vi "TestDBCommands.vi"() -> ()   [LabVIEW 2012]
uses:
  <vilib>/addons/database/Connection.llb/DB Tools Open Connec (Path).vi
  <vilib>/addons/database/Connection.llb/Conn Execute.vi
  <vilib>/addons/database/Recordset.llb/Rec Fetch Recordset Data (R).vi
  <vilib>/addons/database/Recordset.llb/Rec Destroy - Connection.vi
  <vilib>/addons/database/Auxilliary.llb/DB Tools Parameter Dir.ctl
  <vilib>/addons/database/NI_Database_API.lvlib
  <vilib>/addons/database/Auxilliary.llb/DB Tools DataTypes.ctl
  <vilib>/addons/database/Auxilliary.llb/DB Tools Parameter Info.ctl
  <vilib>/addons/database/Command.llb/Cmd Set Parameter Value (C).vi
  <vilib>/addons/database/Command.llb/Cmd Execute.vi
  <vilib>/addons/database/Recordset.llb/Rec Destroy - Command.vi
  <vilib>/addons/database/Command.llb/Cmd Delete.vi
  Controls/ProbeStationId.vi
panel:
  out "SameId?":bool
  out "Tested?":bool
  out "Exists?":bool
  in  "Type":string
  out "String":string
  out "error out":errorcluster
  in  "WaferId":string
  in  "connection":path
  in  "error IO":errorcluster
  out "System":string
  out "Run Number":string
  out "Pocket":string
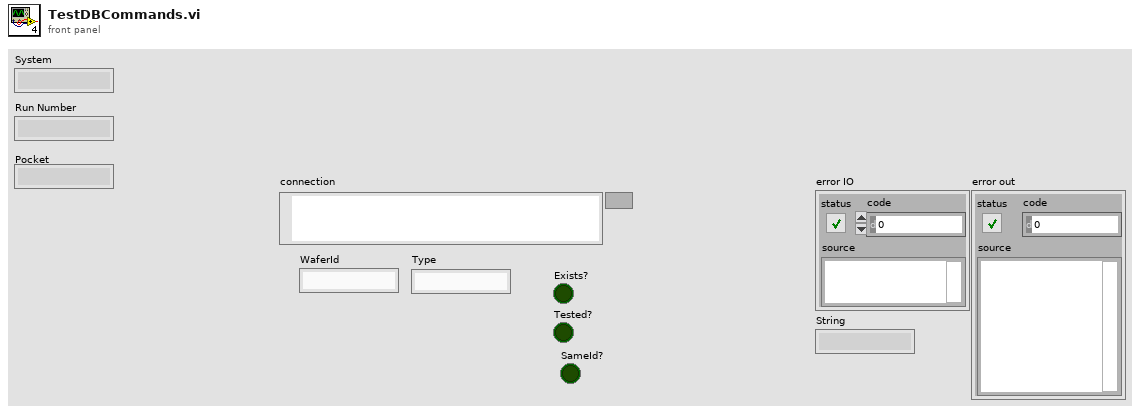
[diagram p1: front panel]
types:
  T1 = typedef "NI_Database_API.lvlib/DB Tools Parameter Info.ctl" = cluster{"parameter name":string, "type":T2, "direction":T3, "value":variant}
  T2 = typedef "NI_Database_API.lvlib/DB Tools DataTypes.ctl" = enum16{"String", "Long (I32)", "Single (SGL)", "Double (DBL)", "Date/Time", "Binary"}
  T3 = typedef "NI_Database_API.lvlib/DB Tools Parameter Dir.ctl" = enum32{"Input", "Output", "Input/Output", "Return Value"}
  T4 = typedef "NI_Database_API.lvlib/Conn ObjectReference.ctl" = refnum<k1>
  T5 = typedef "NI_Database_API.lvlib/Cmd ObjectReference.ctl" = refnum<k1>
  T6 = typedef "NI_Database_API.lvlib/Cmd-Rec Object Reference.ctl" = refnum<k1>
  T7 = typedef "NI_Database_API.lvlib/Rec ObjectReference.ctl" = refnum<k1>
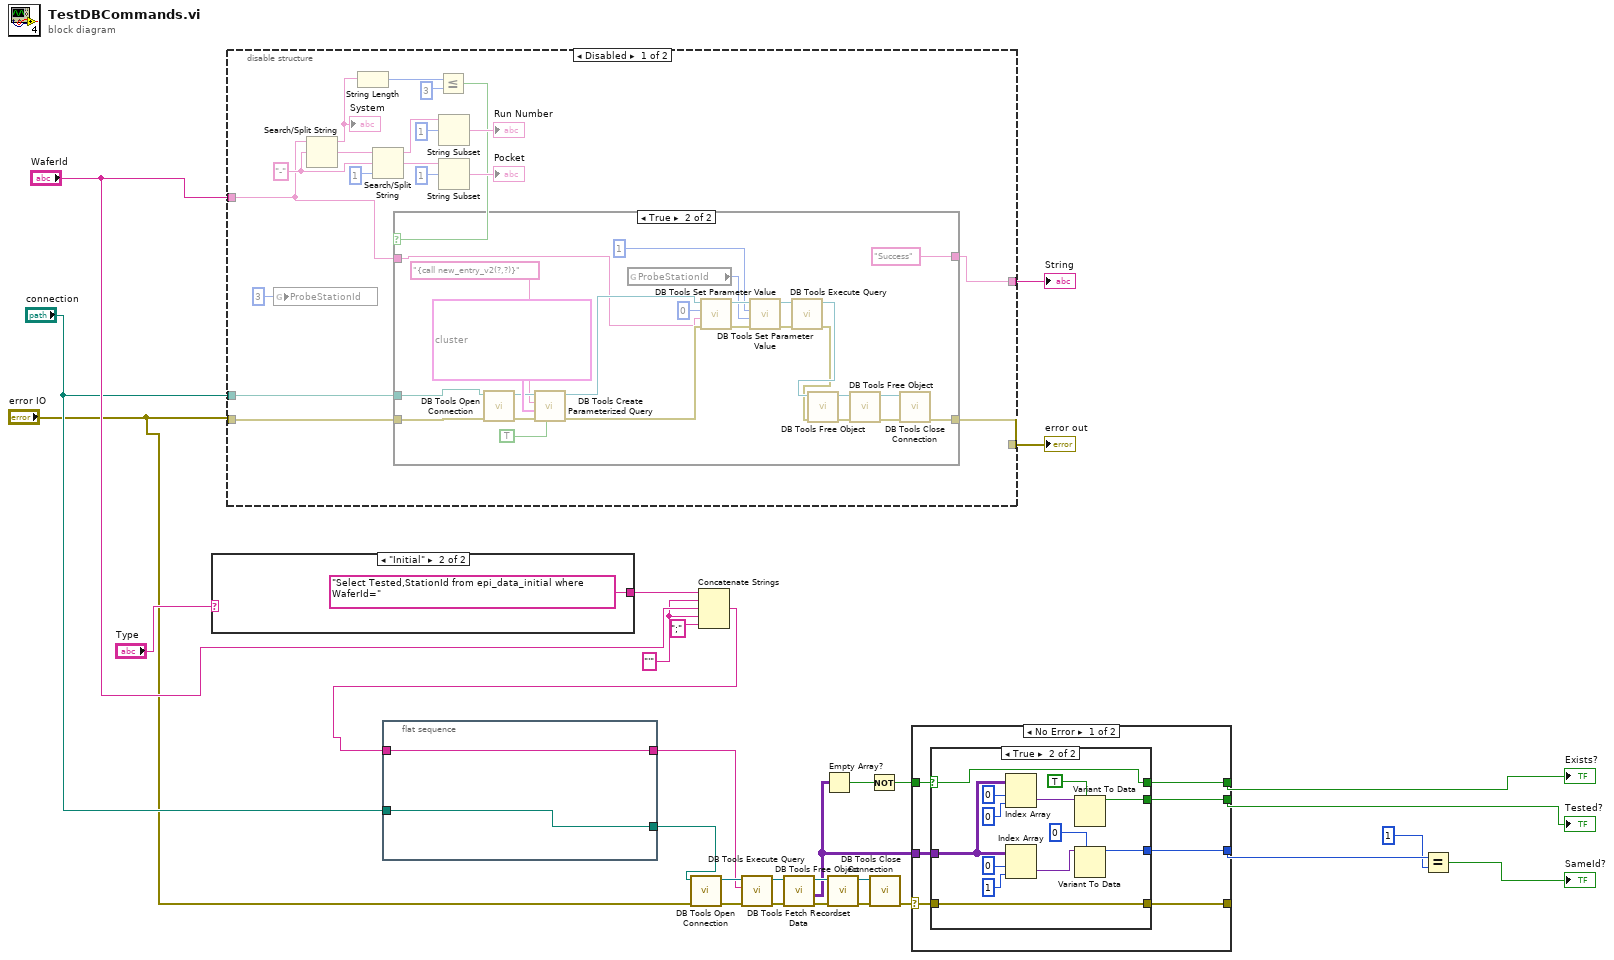
[diagram p0: block diagram]
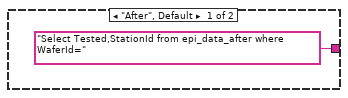
[diagram p2: hidden frame]
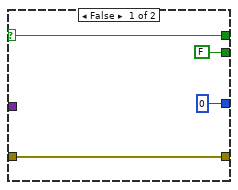
[diagram p3: hidden frame]
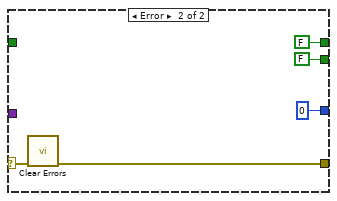
[diagram p4: hidden frame]
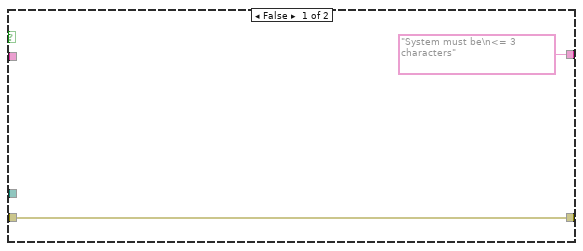
[diagram p5: hidden frame]
diagram:
  w25 = "'" ("string")
  n1 = case shown="\"Initial\"" "Type" {
    tunnel: ["Select Tested,StationId from epi_data_after where WaferId=" ("string") "Select Tested,StationId from epi_data_initial where WaferId=" ("string")] -> w10
    frame "After", Default {
    }
    frame "Initial" {
    }
  }
  n2 = disable-structure shown="Disabled" {
    disable-tunnel: [w37 _] -> w29
    disable-tunnel: [w36 _] -> w28
    disable-tunnel: "error IO" -> [w35 _]
    disable-tunnel: "connection" -> [w34 _]
    disable-tunnel: "WaferId" -> [w33 _]
    frame Disabled {
      w49 = "-" ("search string/char (-)")
      n3 = global write "ProbeStationId.vi" "ProbeStationId"(3 ("ProbeStationId")) -> ()
      n4 = Search/Split String(string=w33, search string/char (-)=w49) -> (substring before match=w41:string, match + rest of string=w50:string)  [unwired: 1 in, 1 out]
      "System" <- w41
      n5 = String Length(string=w41) -> (length=w40:i32)
      n6 = Search/Split String(string=w50, search string/char (-)=w49, offset (0)=1) -> (substring before match=w44:string, match + rest of string=w47:string)  [unwired: 1 out]
      n7 = Less Or Equal?(x=w40, y=3) -> (x <= y?=w38:bool)
      n8 = case shown="True" w38 {
        tunnel: w33 -> [_ w56]
        tunnel: [w52 w69] -> w37
        tunnel: w35 -> [w52 w64]
        tunnel: ["System must be\n<= 3 characters" "Success"] -> w36
        tunnel: w34 -> [_ w53]
        frame False {
        }
        frame True {
          n9 = call-poly <vilib>:"DB Tools Open Connection.vi"("error in (no error)"=w64, "connection information"=w53) -> ("error out"=w74:errorcluster, "connection reference"=w75:T4)  [unwired: 6 in]
          n10 = call <vilib>:"DB Tools Create Parameterized Query.vi"("stored procedure? (F)"=TRUE, "error in (no error)"=w74, "parameters"=T1[] [{"parameter name"="wafer", "type"=enum."String", "direction"=enum."Input", "value"=variant}, {"parameter name"="stationId", "type"=enum."Long (I32)", "direction"=enum."Input", "value"=variant}], "SQL query"="{call new_entry_v2(?,?)}", "connection reference"=w75) -> ("error out"=w72:errorcluster, "command reference"=w71:T5)  [unwired: 2 in, 1 out]
          n11 = global read "ProbeStationId.vi" "ProbeStationId"() -> (w55:i32)
          n12 = call-poly <vilib>:"DB Tools Set Parameter Value.vi"("error in (no error)"=w72, "value"=w56, "parameter index"=0, "command reference"=w71) -> ("error out"=w59:errorcluster, "command reference out"=w60:T5)  [unwired: 4 in]
          n13 = call-poly <vilib>:"DB Tools Set Parameter Value.vi"("error in (no error)"=w59, "value"=w55, "parameter index"=1, "command reference"=w60) -> ("error out"=w58:errorcluster, "command reference out"=w57:T5)  [unwired: 4 in]
          n14 = call-poly <vilib>:"DB Tools Execute Query.vi"("error in (no error)"=w58, "command reference"=w57) -> ("error out"=w67:errorcluster, "command-recordset reference"=w68:T6)  [unwired: 6 in]
          n15 = call-poly <vilib>:"DB Tools Free Object.vi"("error in (no error)"=w67, "command-recordset reference"=w68) -> ("error out"=w70:errorcluster, "command reference"=w61:T5)  [unwired: 8 in]
          n16 = call-poly <vilib>:"DB Tools Free Object.vi"("error in (no error)"=w70, "command reference"=w61) -> ("error out"=w65:errorcluster, "connection reference"=w66:T4)  [unwired: 8 in]
          n17 = call <vilib>:"DB Tools Close Connection.vi"("error in (no error)"=w65, "connection reference"=w66) -> ("error out"=w69:errorcluster)  [unwired: 5 in]
        }
      }
      n18 = String Subset(string=w44, offset (0)=1) -> (substring=→"Run Number":string)  [unwired: 1 in]
      n19 = String Subset(string=w47, offset (0)=1) -> (substring=→"Pocket":string)  [unwired: 1 in]
    }
    frame Enabled {
    }
  }
  "error out" <- w29
  "String" <- w28
  n20 = flat-sequence {
    tunnel: [w79] -> w2
    tunnel: w6 -> [w79]
    tunnel: [w78] -> w5
    tunnel: "connection" -> [w78]
    frame #0 {
    }
  }
  n21 = call-poly <vilib>:"DB Tools Open Connection.vi"("error in (no error)"="error IO", "connection information"=w5) -> ("error out"=w22:errorcluster, "connection reference"=w23:T4)  [unwired: 6 in]
  n22 = Concatenate Strings(w10, w25, "WaferId", w25, ";" ("string")) -> (w6:string)
  n23 = call-poly <vilib>:"DB Tools Execute Query.vi"("error in (no error)"=w22, "SQL query"=w2, "connection reference"=w23) -> ("error out"=w18:errorcluster, "recordset reference"=w19:T7)  [unwired: 5 in]
  n24 = call-poly <vilib>:"DB Tools Fetch Recordset Data.vi"("error in (no error)"=w18, "recordset reference"=w19) -> ("error out"=w16:errorcluster, "recordset data"=w12:variant[][], "recordset reference out"=w17:T7)  [unwired: 3 in]
  n25 = Empty Array?(array=w12) -> (empty?=w15:bool)
  n26 = call-poly <vilib>:"DB Tools Free Object.vi"("error in (no error)"=w16, "recordset reference"=w17) -> ("error out"=w20:errorcluster, "connection reference"=w21:T4)  [unwired: 8 in]
  n27 = Not(x=w15) -> (.not. x?=w13:bool)
  n28 = call <vilib>:"DB Tools Close Connection.vi"("error in (no error)"=w20, "connection reference"=w21) -> ("error out"=w14:errorcluster)  [unwired: 5 in]
  n29 = case shown="No Error" w14 {
    selector: w14 -> [w83 w108]
    tunnel: w13 -> [w86 _]
    tunnel: [w84 w107] -> _
    tunnel: w12 -> [w85 _]
    tunnel: [w82 FALSE] -> w8
    tunnel: [w81 FALSE] -> w9
    tunnel: [w80 0] -> w11
    frame No Error {
      n30 = case shown="True" w86 {
        selector: w86 -> [w88 w103]
        tunnel: w85 -> [_ w95]
        tunnel: [w90 w96] -> w84
        tunnel: w83 -> [w90 w96]
        tunnel: [FALSE w92] -> w82
        tunnel: [w88 w103] -> w81
        tunnel: [0 w91] -> w80
        frame False {
        }
        frame True {
          n31 = Index Array(array=w95, index (row)=0, index (col)=0 ("disabled index (col)")) -> (element=w100:variant)
          n32 = Index Array(array=w95, index (row)=0, index (col)=1 ("disabled index (col)")) -> (element=w97:variant)
          n33 = Variant To Data(type=TRUE, Variant=w100) -> (data=w92:bool)  [unwired: 1 in, 1 out]
          n34 = Variant To Data(type=0, Variant=w97) -> (data=w91:i32)  [unwired: 1 in, 1 out]
        }
      }
    }
    frame Error {
      n35 = call <vilib>:"Clear Errors.vi"("error in (no error)"=w108) -> ("error out"=w107:errorcluster)  [unwired: 6 in]
    }
  }
  "Exists?" <- w9
  "Tested?" <- w8
  n36 = Equal?(x=w11, y=1 ("ProbeStationId")) -> (x = y?=→"SameId?":bool)
